vi "Vacuum Test - Step 4.vi"(7 "Step":i32, 8 "error in":errorcluster, 9 "Test Results":T9, 10 "Oil In":T1, 11 "Test Configuration":T2) -> (0 "error out":errorcluster, 1 "Test Results Out":T9, 2 "Oil Out":T1, 3 "Test Configuration Out":T2)   [LabVIEW 2015]
uses:
  Controls/Test Results.ctl
  Controls/Step Result.ctl
  Controls/Startup Test.ctl
  Controls/Test Information.ctl
  Controls/Vacuum Test.ctl
  Controls/Test Timing.ctl
  Controls/Vaccum Thresholds.ctl
  Controls/Helium Test.ctl
  Controls/Helium Thresholds.ctl
  Controls/Startup Thresholds.ctl
  CAN Communication/Oil/Typedefs/Session Handle.ctl
  CAN Communication/Oil/Oil.lvclass
panel:
  out "NI-DAQ Pressure":dbl
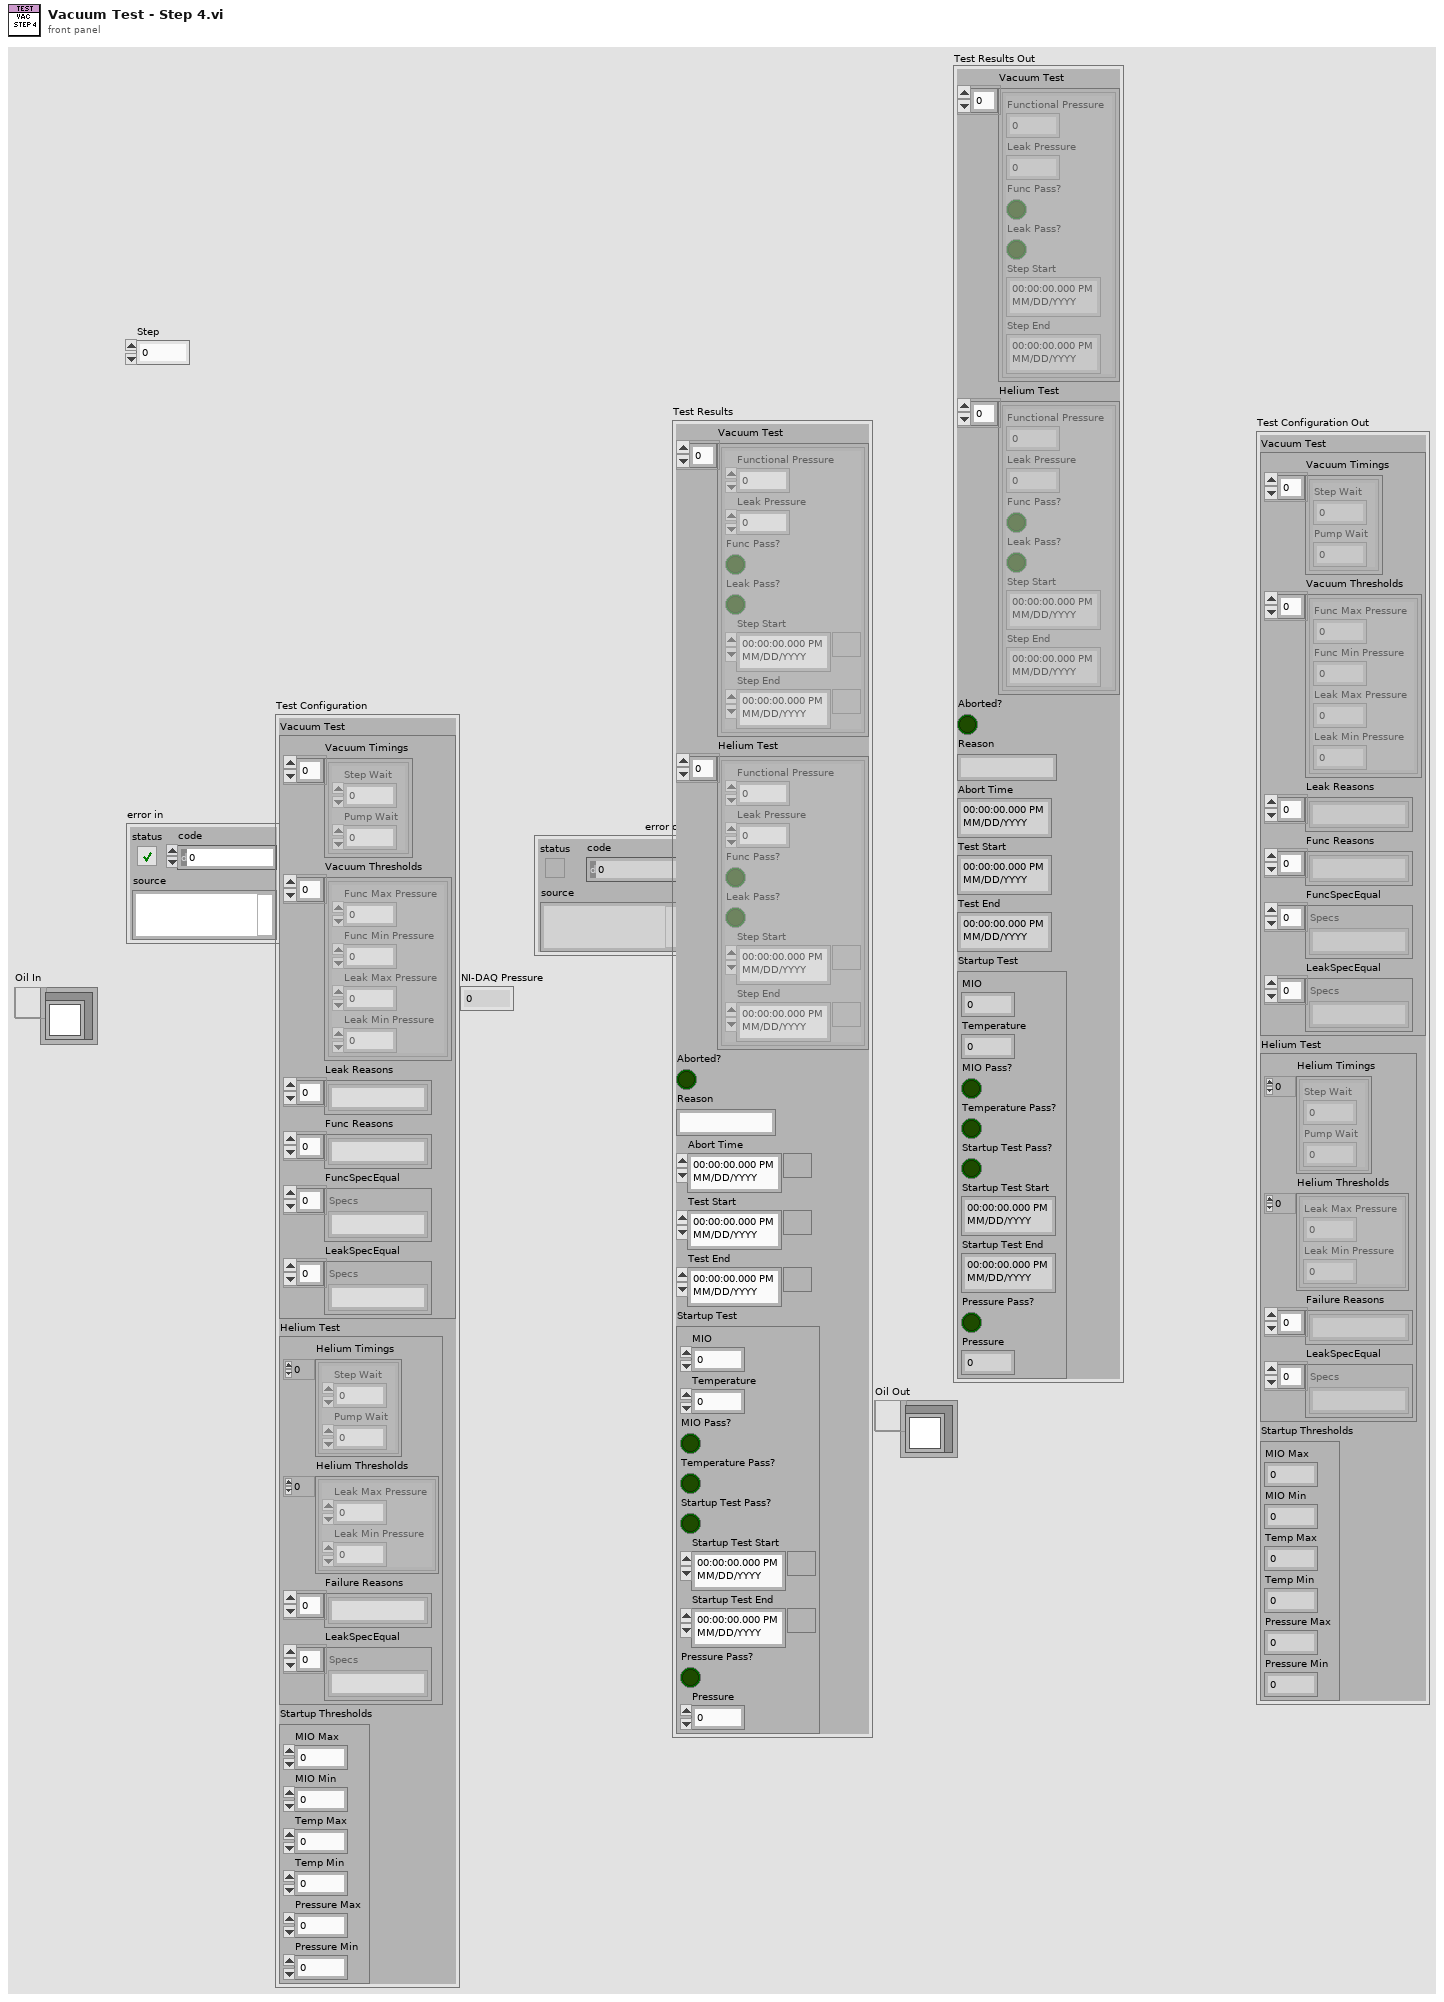
[diagram p1: front panel]
types:
  T1 = typedef "Oil.lvclass/Session Handle.ctl" = refnum<data-value>
  T2 = typedef "Test Information.ctl" = cluster{"Vacuum Test":T3, "Helium Test":T6, "Startup Thresholds":T8}
  T3 = typedef "Vacuum Test.ctl" = cluster{"Vacuum Timings":T4[], "Vacuum Thresholds":T5[], "Leak Reasons":string[], "Func Reasons":string[], "FuncSpecEqual":string[], "LeakSpecEqual":string[]}
  T4 = typedef "Test Timing.ctl" = cluster{"Step Wait":dbl, "Pump Wait":dbl}
  T5 = typedef "Vaccum Thresholds.ctl" = cluster{"Func Max Pressure":dbl, "Func Min Pressure":dbl, "Leak Max Pressure":dbl, "Leak Min Pressure":dbl}
  T6 = typedef "Helium Test.ctl" = cluster{"Helium Timings":T4[], "Helium Thresholds":T7[], "Failure Reasons":string[], "LeakSpecEqual":string[]}
  T7 = typedef "Helium Thresholds.ctl" = cluster{"Leak Max Pressure":dbl, "Leak Min Pressure":dbl}
  T8 = typedef "Startup Thresholds.ctl" = cluster{"MIO Max":dbl, "MIO Min":dbl, "Temp Max":dbl, "Temp Min":dbl, "Pressure Max":dbl, "Pressure Min":dbl}
  T9 = typedef "Test Results.ctl" = cluster{"Vacuum Test":T10[], "Helium Test":T10[], "Aborted?":bool, "Reason":string, "Abort Time":timestamp, "Test Start":timestamp, "Test End":timestamp, "Startup Test":T11}
  T10 = typedef "Step Result.ctl" = cluster{"Functional Pressure":dbl, "Leak Pressure":dbl, "Func Pass?":bool, "Leak Pass?":bool, "Step Start":timestamp, "Step End":timestamp}
  T11 = typedef "Startup Test.ctl" = cluster{"MIO":dbl, "Temperature":dbl, "MIO Pass?":bool, "Temperature Pass?":bool, "Startup Test Pass?":bool, "Startup Test Start":timestamp, "Startup Test End":timestamp, "Pressure Pass?":bool, "Pressure":dbl}
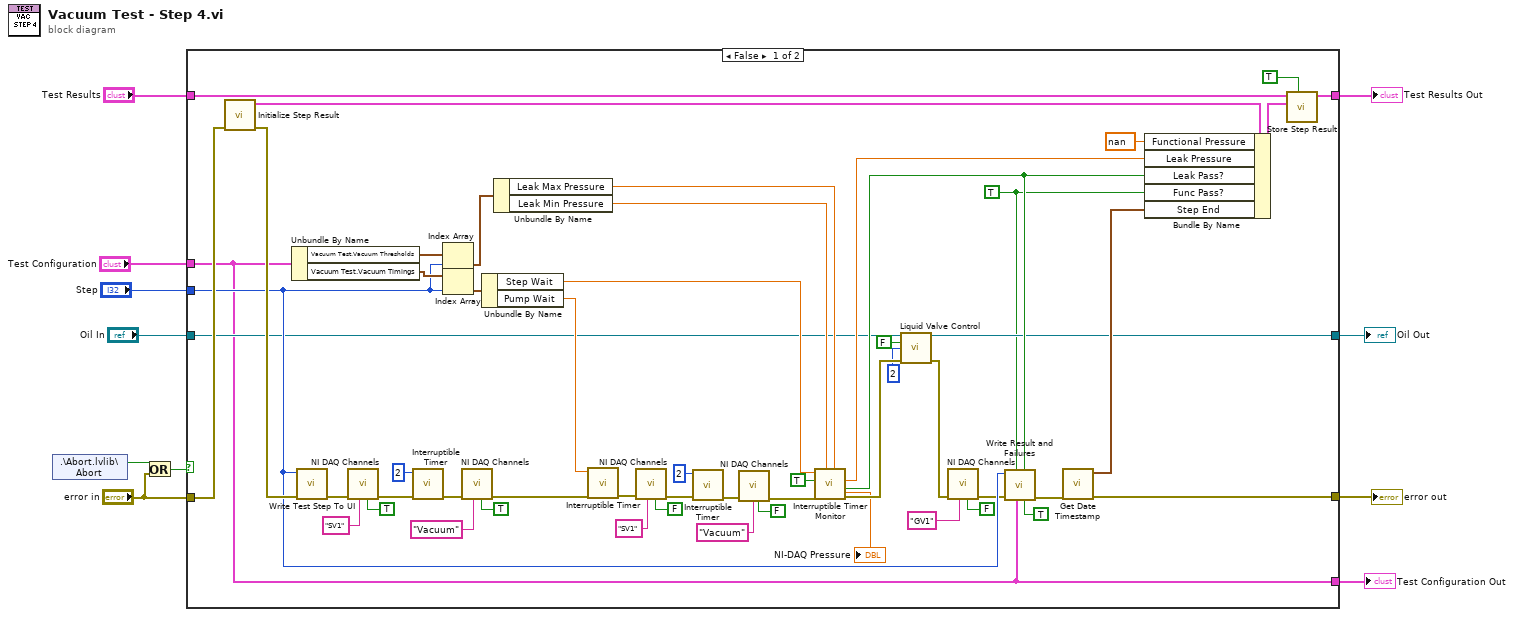
[diagram p0: block diagram]
diagram:
  n1 = shared-variable ".\\Abort.lvlib\\Abort"() -> (w10:bool)  [unwired: 1 in, 1 out]
  n2 = Or(x=w10, y="error in") -> (x .or. y?=w9:bool)
  n3 = case shown="False" w9 {
    tunnel: "error in" -> [w65 w68]
    tunnel: "Test Results" -> [w62 w69]
    tunnel: [w63 w69] -> w8
    tunnel: [w32 w68] -> w7
    tunnel: "Test Configuration" -> [w19 w67]
    tunnel: "Step" -> [w51 _]
    tunnel: [w19 w67] -> w3
    tunnel: [w22 w66] -> w1
    tunnel: "Oil In" -> [w29 w66]
    frame False {
      w21 = TRUE ("Func Pass?")
      n4 = call "Initialize Step Result.vi"("error in (no error)"=w65) -> ("error out"=w64:errorcluster, "New Step Result"=w61:T10)  [unwired: 8 in, 1 out]
      n5 = Unbundle By Name(w19) -> ("Vacuum Test.Vacuum Thresholds"=w58:T5[], "Vacuum Test.Vacuum Timings"=w57:T4[])
      n6 = call "Write Test Step To UI.vi"("error in (no error)"=w64, "Step"=w51) -> ("error out"=w49:errorcluster)  [unwired: 9 in]
      n7 = call "NI DAQ Channels.vi"("Control"=TRUE ("State"), "Channel"="SV1", "error in (no error)"=w49) -> ("error out"=w48:errorcluster)  [unwired: 7 in, 1 out]
      n8 = call "Interruptible Timer.vi"("error in (no error)"=w48, "Wait (s)"=2) -> ("error out"=w31:errorcluster)  [unwired: 7 in, 2 out]
      n9 = Index Array(array=w58, index=w51) -> (element=w53:T5)
      n10 = Index Array(array=w57, index=w51) -> (element=w56:T4)
      n11 = call "NI DAQ Channels.vi"("Control"=TRUE ("State"), "Channel"="Vacuum", "error in (no error)"=w31) -> ("error out"=w43:errorcluster)  [unwired: 7 in, 1 out]
      n12 = Unbundle By Name(w56) -> ("Step Wait"=w39:dbl, "Pump Wait"=w54:dbl)
      n13 = Unbundle By Name(w53) -> ("Leak Max Pressure"=w36:dbl, "Leak Min Pressure"=w37:dbl)
      n14 = call "Interruptible Timer.vi"("error in (no error)"=w43, "Wait (s)"=w54) -> ("error out"=w30:errorcluster)  [unwired: 7 in, 2 out]
      n15 = call "NI DAQ Channels.vi"("Control"=FALSE ("State"), "Channel"="SV1", "error in (no error)"=w30) -> ("error out"=w45:errorcluster)  [unwired: 7 in, 1 out]
      n16 = call "Interruptible Timer.vi"("error in (no error)"=w45, "Wait (s)"=2) -> ("error out"=w41:errorcluster)  [unwired: 7 in, 2 out]
      n17 = call "NI DAQ Channels.vi"("Control"=FALSE ("State"), "Channel"="Vacuum", "error in (no error)"=w41) -> ("error out"=w40:errorcluster)  [unwired: 7 in, 1 out]
      n18 = call "Interruptible Timer Monitor.vi"("Max"=w36, "Min"=w37, "error in (no error)"=w40, "Update UI?"=TRUE, "Wait (s)"=w39) -> ("error out"=w28:errorcluster, "In Range?"=w34:bool, "Leak Rate"=w35:dbl, "NI-DAQ Pressure"=→"NI-DAQ Pressure":dbl)  [unwired: 2 in, 1 out]
      n19 = call "Liquid Valve Control.vi"("Session Handle in"=w29, "On?"=FALSE, "Valve"=2, "error in (no error)"=w28) -> ("Session Handle out"=w22:T1, "error out"=w23:errorcluster)  [unwired: 8 in, 2 out]
      n20 = call "NI DAQ Channels.vi"("Control"=FALSE ("State"), "Channel"="GV1", "error in (no error)"=w23) -> ("error out"=w24:errorcluster)  [unwired: 7 in, 1 out]
      n21 = call "Write Result and Failures.vi"("Vacuum?"=TRUE, "Leak"=w34, "Test Configuration"=w19, "Func"=w21, "error in (no error)"=w24, "Step"=w51) -> ("error out"=w33:errorcluster)  [unwired: 5 in]
      n22 = call "Get Date Timestamp.vi"("error in (no error)"=w33) -> ("error out"=w32:errorcluster, "current time"=w59:timestamp)  [unwired: 9 in]
      n23 = Bundle By Name(cluster=w61, "Functional Pressure"=nan, "Leak Pressure"=w35, "Leak Pass?"=w34, "Func Pass?"=w21, "Step End"=w59) -> (w60:T10)
      n24 = call "Store Step Result.vi"("Vacuum?"=TRUE, "Step Result"=w60, "Test Results In"=w62) -> ("Test Results Out"=w63:T9)  [unwired: 8 in]
    }
    frame True {
    }
  }
  "error out" <- w7
  "Test Results Out" <- w8
  "Test Configuration Out" <- w3
  "Oil Out" <- w1
